vi "Manage Background Music.vi"(8 "error in (no error)":errorcluster, 9 "Music Paused":bool, 10 "Dyn Sounds Path":path, 11 "Sounds":T3(array[cluster]) {"Task ID" format="%.0x"}) -> (0 "error out":errorcluster, 3 "Sounds Out":T3(array[cluster]) {"Task ID" format="%.0x"}, 5 "BackGround Track":string)   [LabVIEW 2021]
uses:
  Typedefs/Sound Effects.ctl
  <vilib>/sound2/lvsound2.llb/Sound Output Task ID.ctl
  <vilib>/numeric/Random Number (Range) DBL.vi
  <vilib>/sound2/lvsound2.llb/Sound Output Set Volume (Single).vi
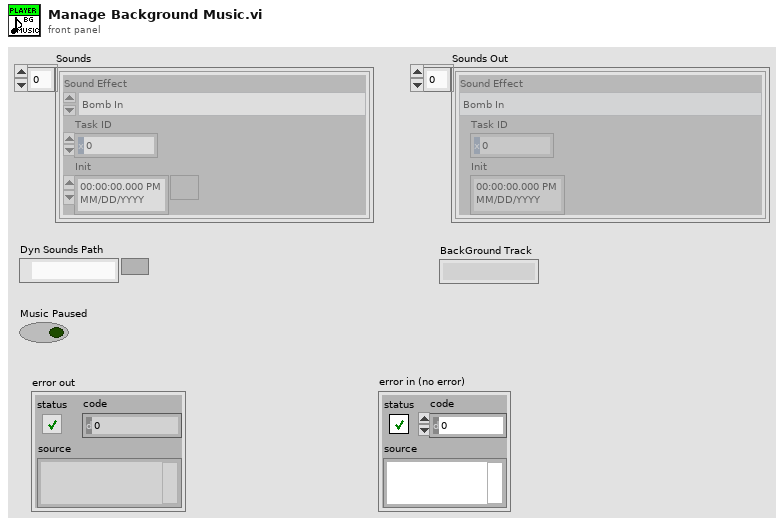
[diagram p1: front panel]
types:
  T1 = typedef "Sound Effects.ctl" = enum16{"Bomb In", "Bomb Out", "Bomb Touched", "Game Over", "Victory", "Eat", "10 Fruits", "Eat2", "Eat3", "Eat4", "MaxShield", "Shield", "10p", "Grape In", "Grape Out", "20p", "30p", "40p", "50p", "60p", "70p", "80p", "90p", "100p", "All shields cracked", "Mouse In", "Mouse Out", "Mouse Eaten", "Grape Eaten", "States Recover", "Broken Shield", "Bonus", "Happy Time", "explode", "Game over musica", "Back Music", "Shield Catch", "Evil lough", "Cricket In", "Cricket eaten", "Lets Go", "Jump1", "Jump2", "Jump3", "Unstoppable", "Troll Music", "winner"}
  T2 = typedef "Sound Output Task ID.ctl" = u32
  T3 = cluster{"Sound Effect":T1, "Task ID":T2, "Init":timestamp}[]
  T4 = cluster{"Sound Effect":T1, "Task ID":T2, "Init":timestamp}
  T5 = cluster{"element":T1, "task ID":T2, "seconds since 1Jan1904":timestamp}
  T6 = cluster{"element":T1, "task ID":T2, "seconds since 1Jan1904":timestamp}[]
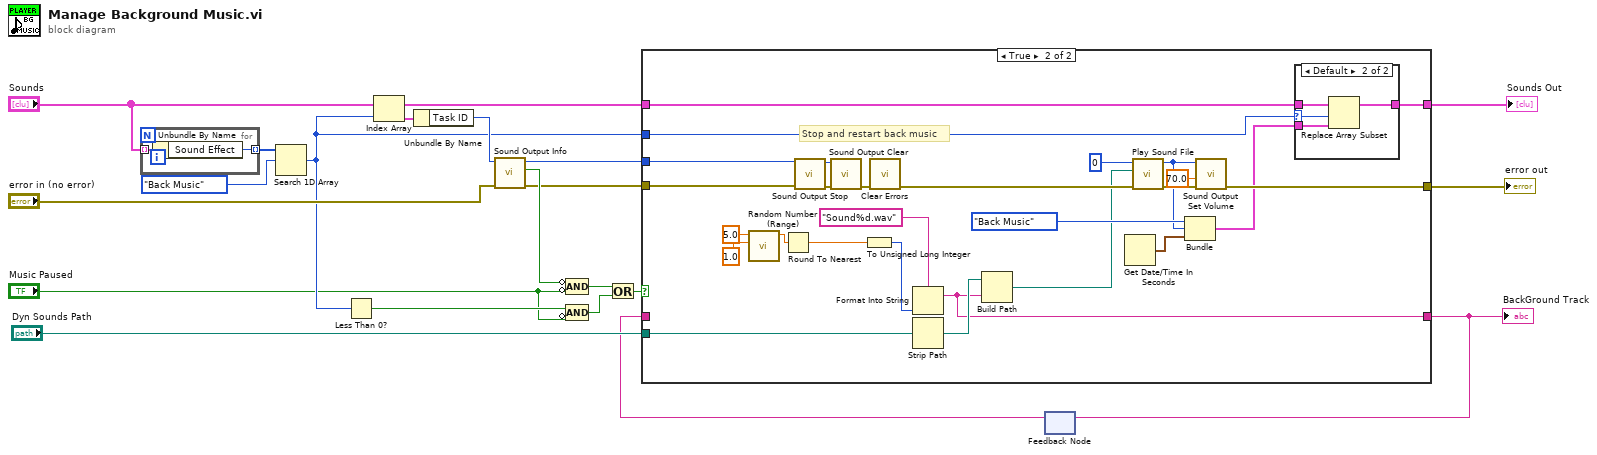
[diagram p0: block diagram]
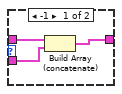
[diagram p3: hidden frame]
diagram:
  n1 = for {
    tunnel: "Sounds" -> [w22] mode=indexing
    tunnel: [w21] -> w17 mode=indexing
    n2 = Unbundle By Name(w22) -> ("Sound Effect"=w21:T1)
  }
  n3 = Search 1D Array(1D array=w17, element=Sound_Effects."Back Music") -> (index of element=w8:i32)  [unwired: 1 in]
  n4 = Less Than 0?(x=w8) -> (x < 0?=w7:bool)
  n5 = Index Array(array="Sounds", index=w8) -> (element=w19:T4)
  n6 = Unbundle By Name(w19) -> ("Task ID"=w20:T2)
  n7 = call <vilib>:"Sound Output Info.vi"("error in (no error)"="error in (no error)", "task ID"=w20) -> ("error out"=w12:errorcluster, "is playing?"=w15:bool, "task ID out"=w13:T2)  [unwired: 6 in, 1 out]
  n8 = Compound Arithmetic op=AND(invert w15, invert "Music Paused") -> (w14:bool)
  n9 = Compound Arithmetic op=AND(w7, invert "Music Paused") -> (w4:bool)
  n10 = Or(x=w14, y=w4) -> (x .or. y?=w5:bool)
  n11 = feedback #1() -> (w1:string)  [unwired: 1 in]
  n12 = case shown="True" w5 {
    tunnel: w13 -> [_ w50]
    tunnel: w12 -> [w24 w49]
    tunnel: "Sounds" -> [w25 w47]
    tunnel: [w24 w41] -> w9
    tunnel: w8 -> [_ w39]
    tunnel: [w25 w38] -> w10
    tunnel: "Dyn Sounds Path" -> [_ w29]
    tunnel: [w23 w27] -> w2
    tunnel: w1 -> [w23 _]
    frame False {
    }
    frame True {
      # "Stop and restart back music"
      n13 = call-poly <vilib>:"Random Number (Range).vi"("lower bound (0)"=1.0 ("Low"), "upper bound (100)"=5.0 ("High")) -> ("number"=w35:dbl)  [unwired: 9 in]
      n14 = Round To Nearest(number=w35) -> (nearest integer value=w34:dbl)
      n15 = call <vilib>:"Sound Output Stop.vi"("error in (no error)"=w49, "task ID"=w50) -> ("error out"=w48:errorcluster, "task ID out"=w51:T2)  [unwired: 8 in]
      n16 = call <vilib>:"Sound Output Clear.vi"("error in (no error)"=w48, "task ID"=w51) -> ("error out"=w52:errorcluster)  [unwired: 9 in]
      n17 = To Unsigned Long Integer(number=w34) -> (unsigned 32bit integer=w32:u32)
      n18 = call <vilib>:"Clear Errors.vi"("error in (no error)"=w52) -> ("error out"=w44:errorcluster)  [unwired: 5 in, 1 out]
      n19 = Format Into String(format string="Sound%d.wav", w32) -> (resulting string=w27:string)  [unwired: 2 in, 1 out]
      n20 = Strip Path(path=w29) -> (stripped path=w30:path)  [unwired: 1 out]
      n21 = Build Path(base path=w30, name or relative path=w27) -> (appended path=w31:path)
      n22 = Get Date/Time In Seconds() -> (seconds since 1Jan1904=w26:timestamp)
      n23 = call <vilib>:"Play Sound File.vi"("error in (no error)"=w44, "path"=w31, "device ID"=u32 0) -> ("error out"=w45:errorcluster, "task ID"=w42:T2)  [unwired: 7 in]
      n24 = Bundle("element"=Sound_Effects."Back Music", "task ID"=w42, "seconds since 1Jan1904"=w26) -> (w40:T5)  [unwired: 1 in]
      n25 = call-poly <vilib>:"Sound Output Set Volume.vi"("error in (no error)"=w45, "volume"=70.0, "task ID"=w42) -> ("error out"=w41:errorcluster)  [unwired: 7 in, 1 out]
      n26 = case shown="Default" w39 {
        selector: w39 -> [_ w57]
        tunnel: w47 -> [w55 w59]
        tunnel: w40 -> [w53 w58]
        tunnel: [w54 w56] -> w38
        frame -1 {
          n27 = Build Array (concatenate)(w55, w53) -> (w54:T6)
        }
        frame Default {
          n28 = Replace Array Subset(array=w59, new element=w58, index=w57) -> (w56:T3)
        }
      }
    }
  }
  "Sounds Out" <- w10
  "error out" <- w9
  "BackGround Track" <- w2
  n29 = feedback-in #1(w2) -> ()
